vi "temp control array generator.vi"(8 "error in (no error)":errorcluster, 10 "Flip Polarity":bool, 11 "T control in":T1={"Starting Value"=20.0, "Step size"=21.0, "Ending Value"=40.0} {"Step size" format="%.2f"; "Ending Value" format="%.2f"; "Starting Value" format="%.2f"}) -> (0 "error out":errorcluster, 1 "N temps":i32, 2 "Temp Values":dbl[](array[numeric]) format="%.2f", 3 "T control out":T1={"Starting Value"=20.0, "Step size"=21.0, "Ending Value"=40.0} {"Step size" format="%.2f"; "Ending Value" format="%.2f"; "Starting Value" format="%.2f"})   [LabVIEW 2014]
doc: "this vi creates an evenly spaced set of values over a defined range\n\nPaul K Dixon\nPhysics 350\nCSUSB Physics"
panel:
  # "Temperature Array Generator"
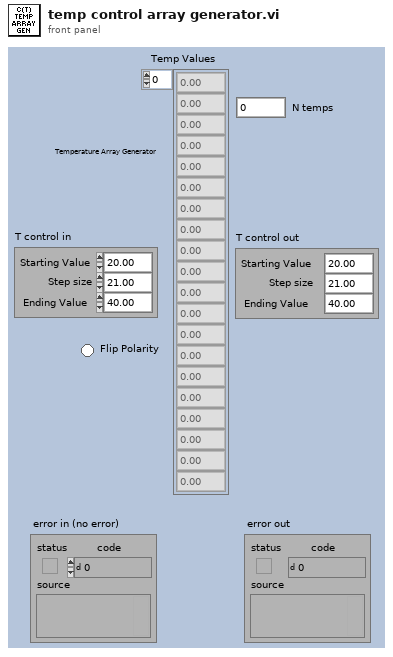
[diagram p1: front panel]
types:
  T1 = cluster{"Starting Value":dbl, "Step size":dbl, "Ending Value":dbl}
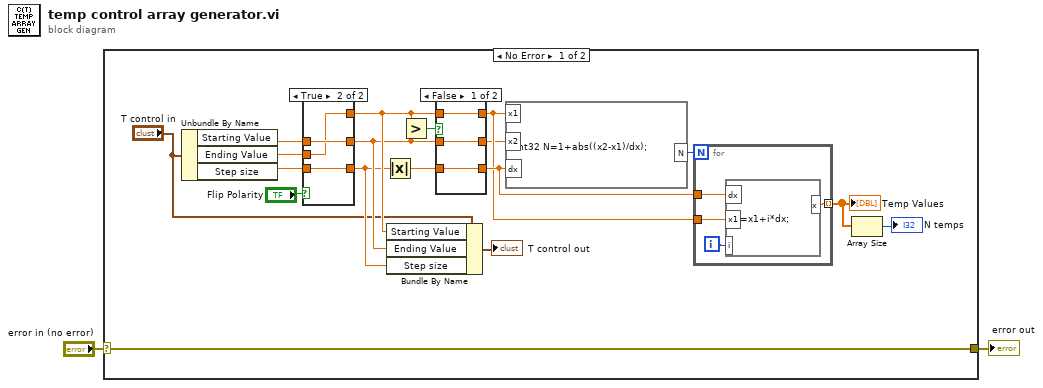
[diagram p0: block diagram]
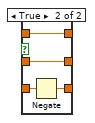
[diagram p3: hidden frame]
diagram:
  n1 = case shown="No Error" "error in (no error)" {
    selector: "error in (no error)" -> [w20 w38]
    tunnel: [w20 w38] -> w1
    frame No Error {
      n2 = Unbundle By Name("T control in") -> ("Starting Value"=w8:dbl, "Ending Value"=w10:dbl, "Step size"=w9:dbl)
      n3 = case shown="True" "Flip Polarity" {
        tunnel: [w23 w24] -> w7
        tunnel: w8 -> [w23 w25]
        tunnel: [w22 w26] -> w5
        tunnel: w9 -> [w22 w26]
        tunnel: [w21 w25] -> w6
        tunnel: w10 -> [w21 w24]
        frame False {
        }
        frame True {
        }
      }
      n4 = Absolute Value(x=w5) -> (abs(x)=w15:dbl)
      n5 = Bundle By Name(cluster="T control in", "Starting Value"=w7, "Ending Value"=w6, "Step size"=w5) -> (→"T control out":T1)
      n6 = Greater?(x=w7, y=w6) -> (0:w18:bool)
      n7 = case shown="False" w18 {
        tunnel: w7 -> [w29 w30]
        tunnel: w6 -> [w28 w31]
        tunnel: [w29 w30] -> w14
        tunnel: [w28 w31] -> w13
        tunnel: w15 -> [w27 w33]
        tunnel: [w27 w32] -> w16
        frame False {
        }
        frame True {
          n8 = Negate(x=w33) -> (-x=w32:dbl)
        }
      }
      n9 = formula code="int32 N=1+abs((x2-x1)/dx);"("x1"=w14, "x2"=w13, "dx"=w16) -> ("N"=w19:i32)
      n10 = for {
        N: w19 -> [_]
        tunnel: [w36] -> w12 mode=indexing
        tunnel: w16 -> [w35]
        tunnel: w14 -> [w34]
        i -> [w37]
        n11 = formula code="x=x1+i*dx;"("x1"=w34, "dx"=w35, "i"=w37) -> ("x"=w36:dbl)
      }
      "Temp Values" <- w12
      n12 = Array Size(array=w12) -> (size(s)=→"N temps":i32)
    }
    frame Error {
    }
  }
  "error out" <- w1
